vi "TEST_CONECTION.vi"(8 "error in (no error)":errorcluster, 10 "password":string, 11 "userID":string) -> (2 "Test Connection":bool)   [LabVIEW 2019, in "DB_VENDING MACHINE.lvlib"]
uses:
  DB_VENDING MACHINE.lvlib
  <vilib>/addons/database/NI_Database_API.lvlib
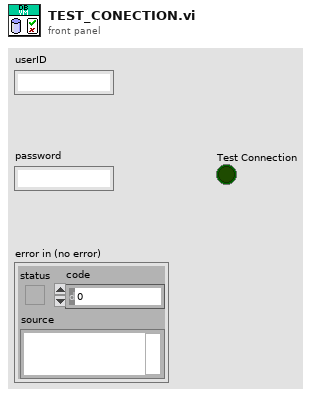
[diagram p1: front panel]
types:
  T1 = typedef "NI_Database_API.lvlib/Conn ObjectReference.ctl" = refnum<k1>
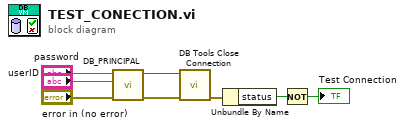
[diagram p0: block diagram]
diagram:
  n1 = call "DB_PRINCIPAL.vi"("error in (no error)"="error in (no error)", "password"="password", "userID"="userID") -> ("error out"=w2:errorcluster, "connection reference"=w1:T1)  [unwired: 7 in]
  n2 = call <vilib>:"DB Tools Close Connection.vi"("error in (no error)"=w2, "connection reference"=w1) -> ("error out"=w8:errorcluster)  [unwired: 5 in]
  n3 = Unbundle By Name(w8) -> ("status"=w7:bool)
  n4 = Not(x=w7) -> (.not. x?=→"Test Connection":bool)
